vi "CalculateModeArray.vi"(8 "General settings":T2, 11 "Holo Control":T1 {"Modes"."Amplititute" step=0.05}) -> (2 "ModeArray":dbl[][](array[numeric]))   [LabVIEW 2014]
uses:
  Controls/SLM General Settings.ctl
  Controls/Holo Controls.ctl
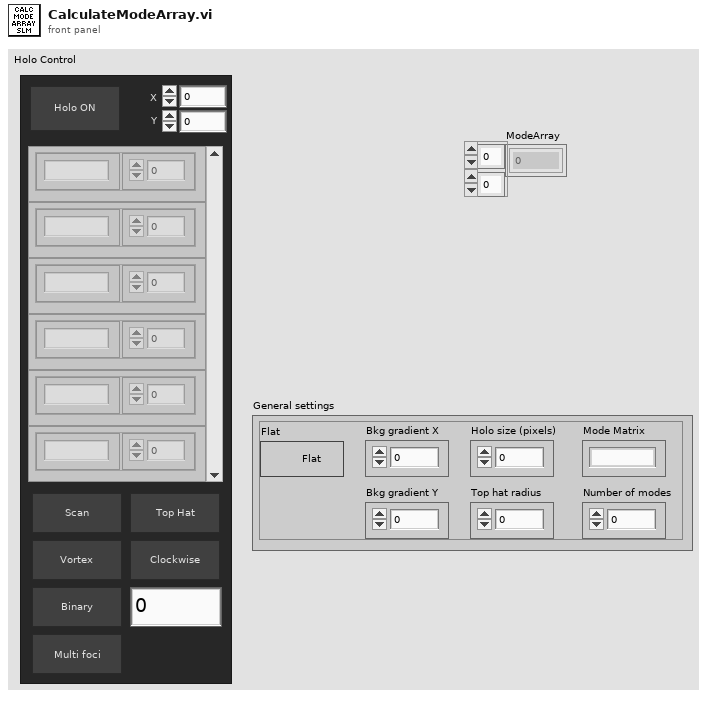
[diagram p1: front panel]
types:
  T1 = typedef "Holo Controls.ctl" = cluster{"Top Hat":bool, "Modes":cluster{"Mode ID":string, "Amplititute":dbl}[], "Vortex":bool, "Clockwise":bool, "X":dbl, "Y":dbl, "Holo ON":bool, "Scan":bool, "Binary":bool, "Binary Angle":dbl, "Multi foci":bool}
  T2 = typedef "SLM General Settings.ctl" = cluster{"Holo size (pixels)":i32, "Top hat radius":dbl, "Number of modes":i32, "Bkg gradient X":dbl, "Bkg gradient Y":dbl, "Flat":bool, "Mode Matrix":u16}
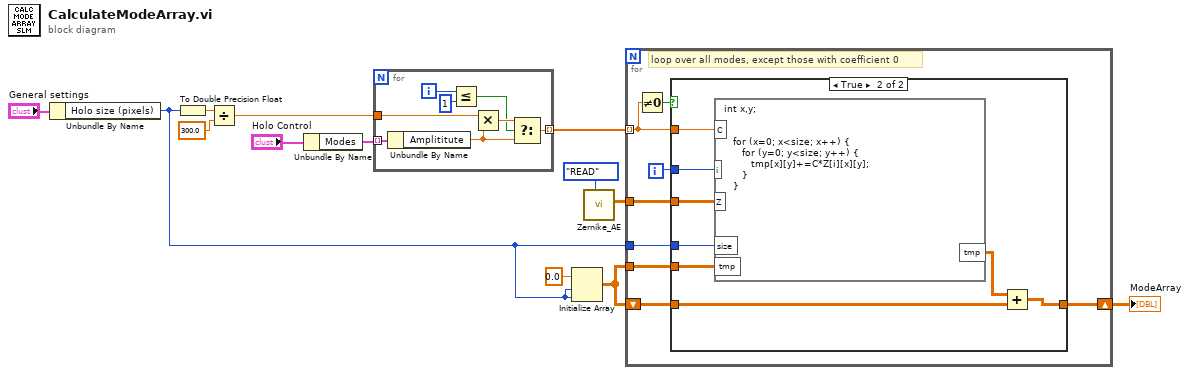
[diagram p0: block diagram]
diagram:
  n1 = Unbundle By Name("General settings") -> ("Holo size (pixels)"=w1:i32)
  n2 = To Double Precision Float(number=w1) -> (double precision float=w6:dbl)
  n3 = Divide(x=w6, y=300.0) -> (x/y=w2:dbl)
  n4 = Unbundle By Name("Holo Control") -> ("Modes"=w4:cluster{"Mode ID":string, "Amplititute":dbl}[])
  n5 = for {
    tunnel: w4 -> [w21] mode=indexing
    tunnel: [w18] -> w3 mode=indexing
    tunnel: w2 -> [w17]
    i -> [w20]
    n6 = Unbundle By Name(w21) -> ("Amplititute"=w16:dbl)
    n7 = Less Or Equal?(x=w20, y=1) -> (x <= y?=w14:bool)
    n8 = Multiply(x=w17, y=w16) -> (x*y=w15:dbl)
    n9 = Select(t=w15, s=w14, f=w16) -> (s? t:f=w18:dbl)
  }
  n10 = Initialize Array(0.0 ("element"), w1, w1) -> (w10:dbl[][])
  n11 = call "Zernike_AE.vi"("Action"=enum16{"READ", "WRITE"}."READ") -> ("Zernike Out"=w8:dbl[][][])  [unwired: 10 in]
  n12 = for {
    shift-right: [w22] -> w12
    shift-left: w10 -> [w23]
    tunnel: w8 -> [w26]
    tunnel: w1 -> [w29]
    tunnel: w3 -> [w25] mode=indexing
    tunnel: w10 -> [w28]
    i -> [w27]
    # "loop over all modes, except those with coefficient 0"
    n13 = Not Equal To 0?(x=w25) -> (x != 0?=w24:bool)
    n14 = case shown="True" w24 {
      tunnel: w29 -> [_ w38]
      tunnel: w28 -> [_ w37]
      tunnel: w25 -> [_ w36]
      tunnel: w27 -> [_ w35]
      tunnel: w26 -> [_ w34]
      tunnel: w23 -> [w30 w32]
      tunnel: [w30 w31] -> w22
      frame False {
      }
      frame True {
        n15 = formula code="int x,y;\n\n\n   for (x=0; x<size; x++) {\n      for (y=0; y<size; y++) {\n         tmp[x][y]+=C*Z[i][x][y];\n      }\n   }"("C"=w36, "size"=w38, "tmp"=w37, "i"=w35, "Z"=w34) -> ("tmp"=w33:dbl[][])
        n16 = Add(x=w33, y=w32) -> (x+y=w31:dbl[][])
      }
    }
  }
  "ModeArray" <- w12
